vi "DBL to FXP Raw.vi"(7 "FXP Configuration":T1, 8 "error in (no error)":errorcluster, 10 "DBL Value":dbl) -> (0 "error out":errorcluster, 2 "Bool Data":bool[](array[boolean]))   [LabVIEW 2026, in "FPGA Register IO.lvlib"]
uses:
  FPGA Register IO.lvlib
  TypeDefs/FXP Configuration.ctl
  <vilib>/fxp/LVFixedPointRepBitsTypeDef.ctl
  <vilib>/fxp/LVFixedPointRepRangeTypeDef.ctl
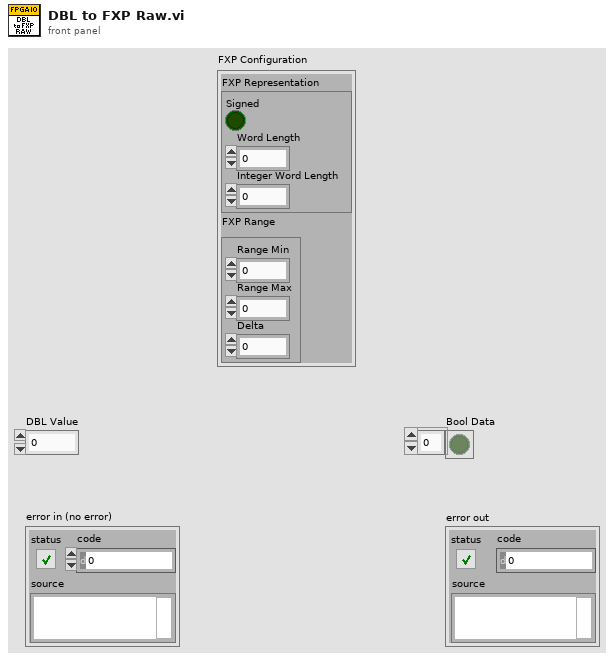
[diagram p1: front panel]
types:
  T1 = typedef "FPGA Register IO.lvlib/FXP Configuration.ctl" = cluster{"FXP Representation":T2, "FXP Range":T3}
  T2 = typedef "LVFixedPointRepBitsTypeDef.ctl" = cluster{"Signed":bool, "Word Length":u32, "Integer Word Length":i32}
  T3 = typedef "LVFixedPointRepRangeTypeDef.ctl" = cluster{"Range Min":dbl, "Range Max":dbl, "Delta":dbl}
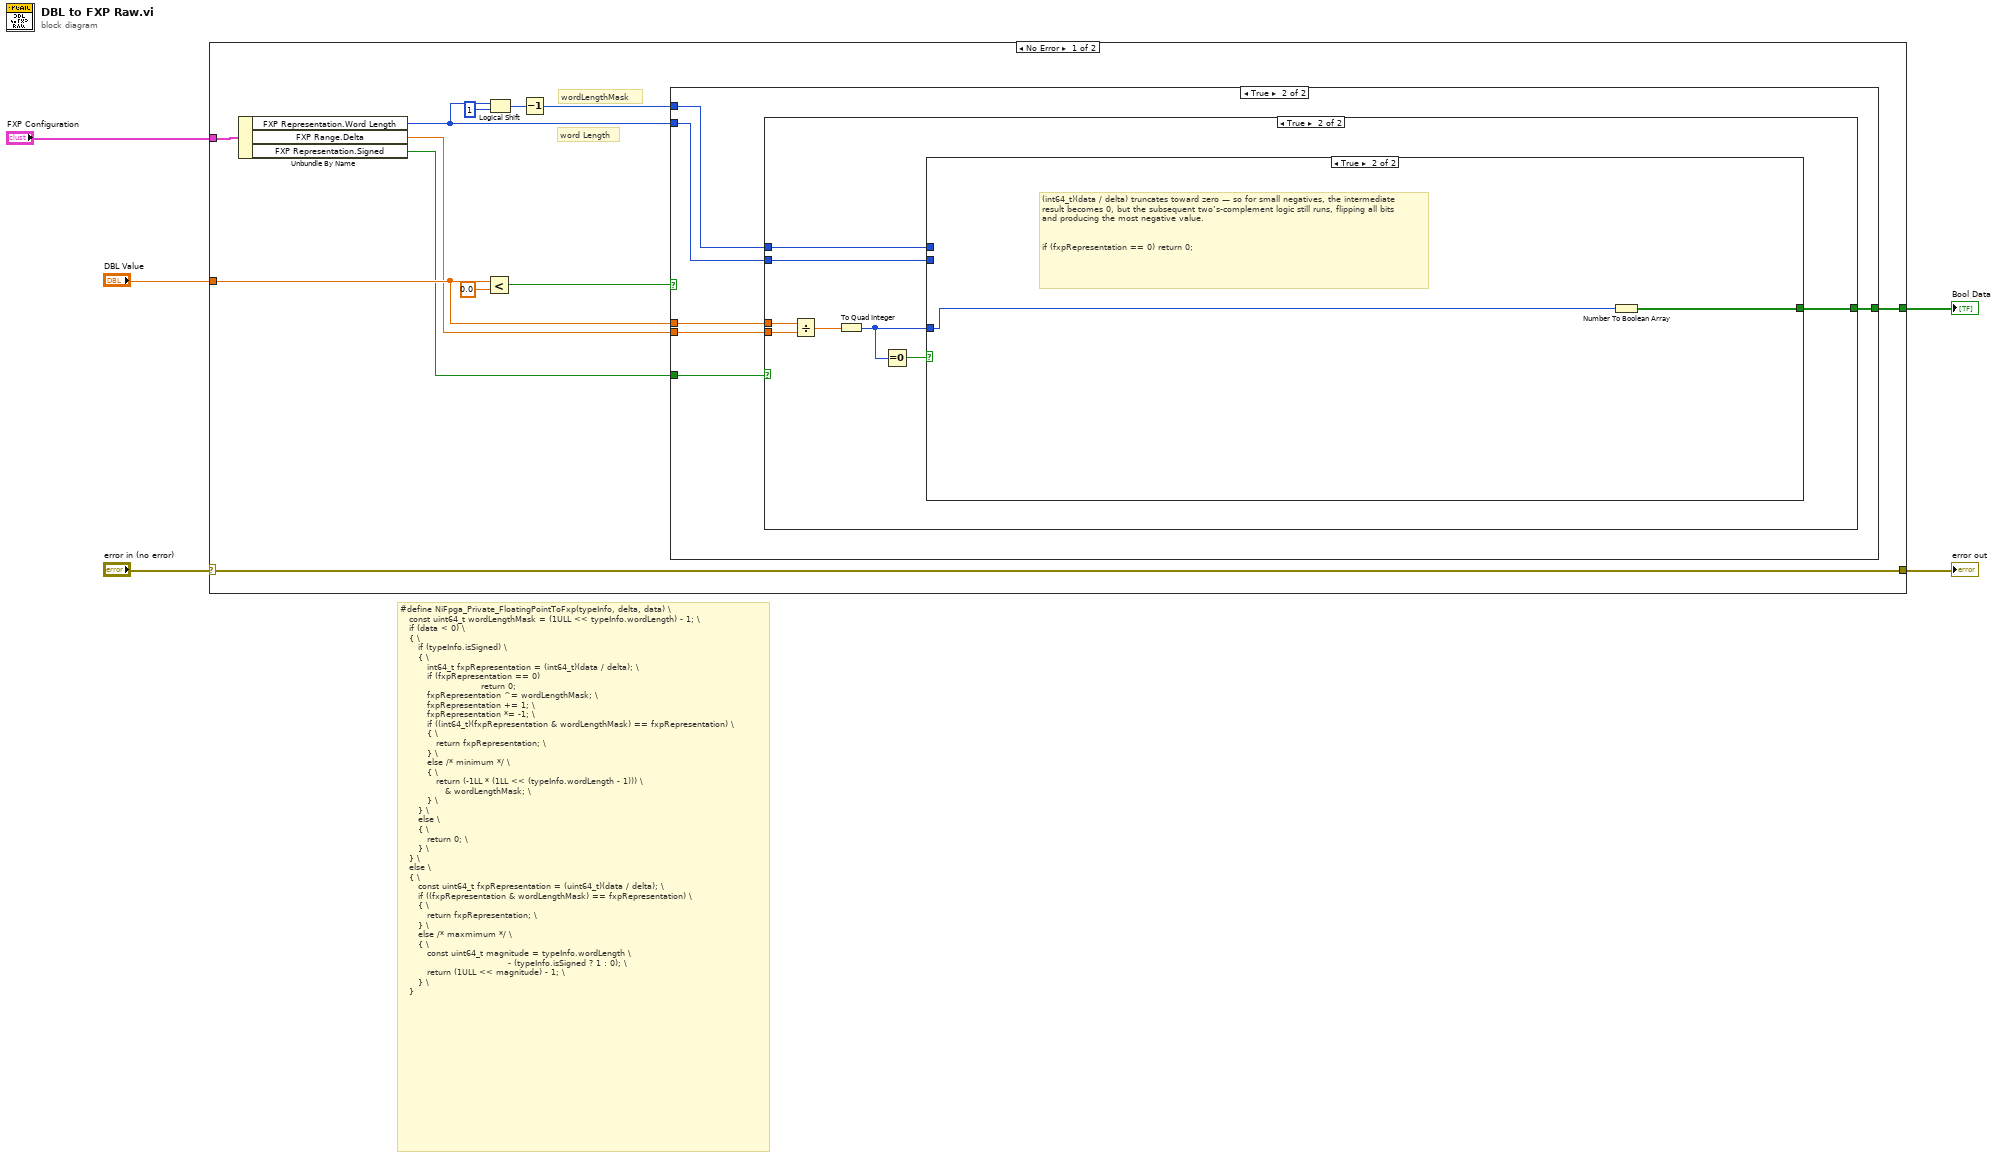
[diagram p0: block diagram]
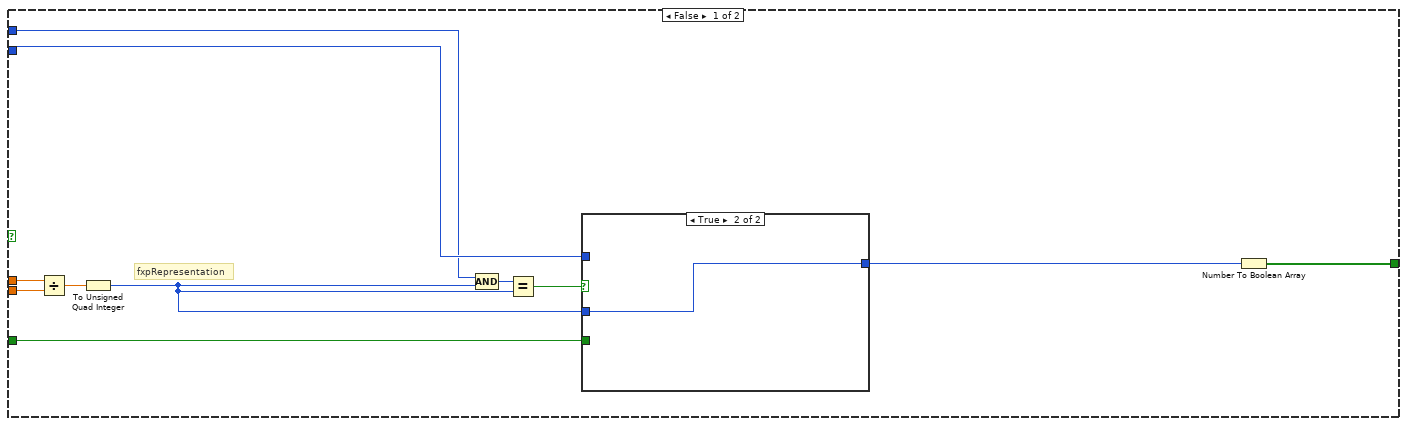
[diagram p2: hidden frame]
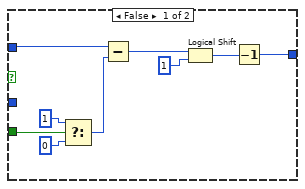
[diagram p3: hidden frame]
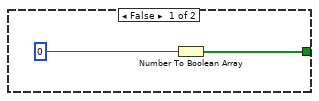
[diagram p4: hidden frame]
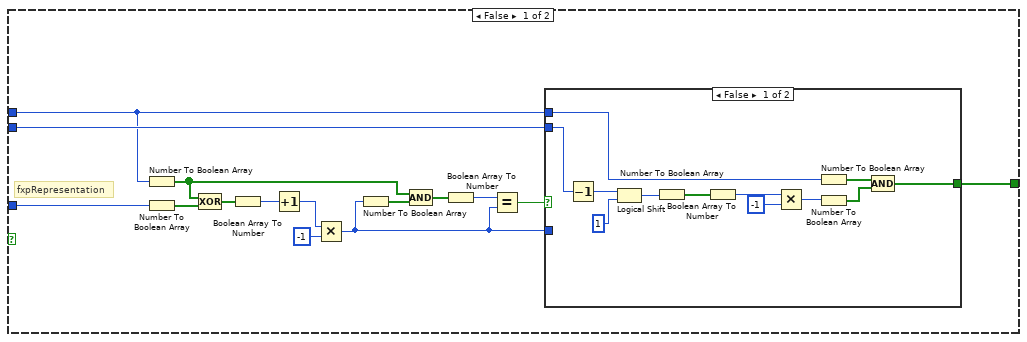
[diagram p5: hidden frame]
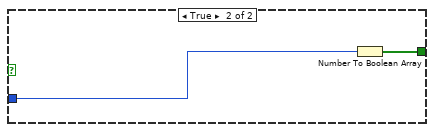
[diagram p6: hidden frame]
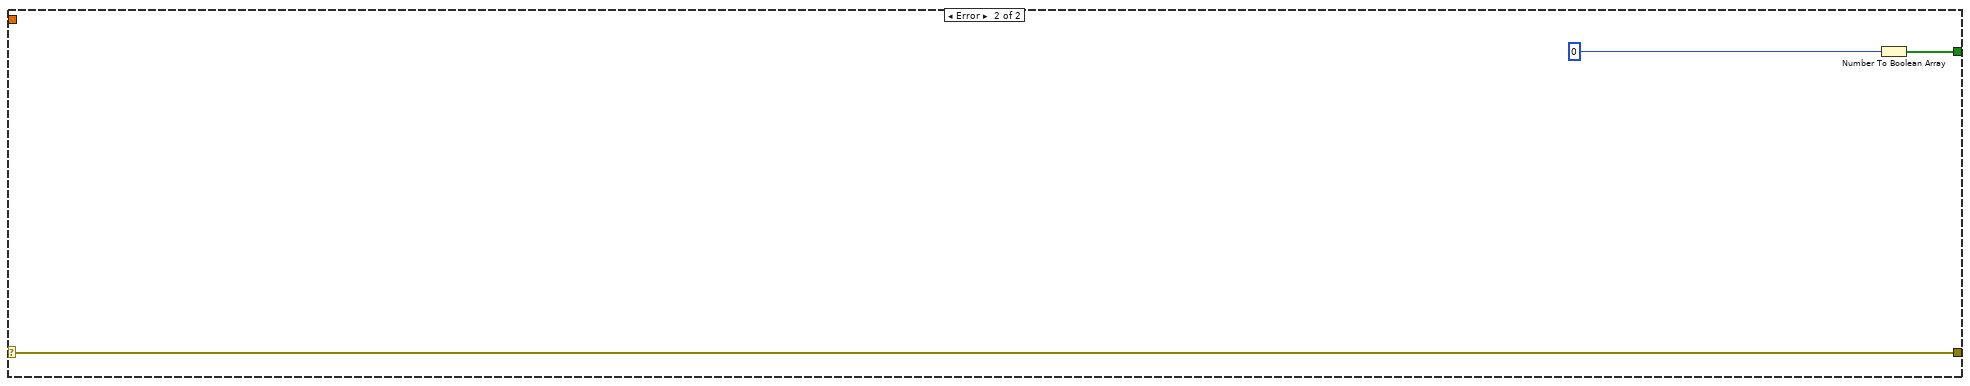
[diagram p7: hidden frame]
diagram:
  # "#define NiFpga_Private_FloatingPointToFxp(typeInfo, delta, data) \\\n   const uint64_t wordLengthMask = (1ULL << typeInfo.wordLength) - 1; \\\n   if (data < 0) \\\n   { \\\n      if (typeInfo.isSigned) \\\n      { \\\n         int64_t fxpRepresentation = (int64_t)(data / delta); \\\n         if (fxpRepresentation == 0)\n                           return 0;\n         fxpRepresentation ^= wordLengthMask; \\\n         fxpRepresentation += 1; \\\n         fxpRepresentation *= -1; \\\n         if ((int64_t)(fxpRepresentation & wordLengthMask) == fxpRepresentation) \\\n         { \\\n            return fxpRepresentation; \\\n         } \\\n         else /* minimum */ \\\n         { \\\n            return (-1LL * (1LL << (typeInfo.wordLength - 1))) \\\n               & wordLengthMask; \\\n         } \\\n      } \\\n      else \\\n      { \\\n         return 0; \\\n      } \\\n   } \\\n   else \\\n   { \\\n      const uint64_t fxpRepresentation = (uint64_t)(data / delta); \\\n      if ((fxpRepresentation & wordLengthMask) == fxpRepresentation) \\\n      { \\\n         return fxpRepresentation; \\\n      } \\\n      else /* maxmimum */ \\\n      { \\\n         const uint64_t magnitude = typeInfo.wordLength \\\n                                    - (typeInfo.isSigned ? 1 : 0); \\\n         return (1ULL << magnitude) - 1; \\\n      } \\\n   }"
  n1 = case shown="No Error" "error in (no error)" {
    selector: "error in (no error)" -> [w8 w88]
    tunnel: "FXP Configuration" -> [w12 _]
    tunnel: [w8 w88] -> w4
    tunnel: "DBL Value" -> [w11 _]
    tunnel: [w7 w87] -> w1
    frame No Error {
      # "word Length"
      # "wordLengthMask"
      n2 = Unbundle By Name(w12) -> ("FXP Representation.Word Length"=w6:u32, "FXP Range.Delta"=w10:dbl, "FXP Representation.Signed"=w9:bool)
      n3 = Less?(x=w11, y=0.0) -> (x < y?=w14:bool)
      n4 = Logical Shift(y=w6, x=u64 1) -> (x << y=w17:u64)
      n5 = Decrement(x=w17) -> (x-1=w13:u64)
      n6 = case shown="True" w14 {
        tunnel: w9 -> [w22 w44]
        tunnel: w11 -> [w28 w43]
        tunnel: w10 -> [w27 w42]
        tunnel: w6 -> [w23 w41]
        tunnel: w13 -> [w21 w40]
        tunnel: [w18 w39] -> w7
        frame False {
          # "fxpRepresentation"
          n7 = Divide(x=w28, y=w27) -> (x/y=w26:dbl)
          n8 = To Unsigned Quad Integer(1:w26) -> (0:w20:u64)
          n9 = Compound Arithmetic op=AND(w21, w20) -> (w25:u64)
          n10 = Equal?(x=w25, y=w20) -> (x = y?=w24:bool)
          n11 = case shown="True" w24 {
            tunnel: [w29 w38] -> w19
            tunnel: w23 -> [w34 _]
            tunnel: w22 -> [w37 _]
            tunnel: w20 -> [_ w38]
            frame False {
              n12 = Select(t=u32 1 ("word length"), s=w37, f=u32 0) -> (s? t:f=w33:u32)
              n13 = Subtract(x=w34, y=w33) -> (x-y=w32:u32)
              n14 = Logical Shift(y=w32, x=u64 1) -> (x << y=w30:u64)
              n15 = Decrement(x=w30) -> (x-1=w29:u64)
            }
            frame True {
            }
          }
          n16 = Number To Boolean Array(number=w19) -> (Boolean array=w18:bool[])
        }
        frame True {
          n17 = case shown="True" w44 {
            tunnel: w43 -> [_ w54]
            tunnel: w42 -> [_ w53]
            tunnel: w40 -> [_ w50]
            tunnel: w41 -> [_ w51]
            tunnel: [w46 w49] -> w39
            frame False {
              n18 = Number To Boolean Array(number=i64 0) -> (Boolean array=w46:bool[])
            }
            frame True {
              n19 = Divide(x=w54, y=w53) -> (x/y=w52:dbl)
              n20 = To Quad Integer(1:w52) -> (0:w48:i64)
              n21 = Equal To 0?(x=w48) -> (x = 0?=w47:bool)
              n22 = case shown="True" w47 {
                tunnel: w48 -> [w69 w85]
                tunnel: w51 -> [w60 _]
                tunnel: w50 -> [w56 _]
                tunnel: [w55 w84] -> w49
                frame False {
                  # "fxpRepresentation"
                  n23 = Number To Boolean Array(number=w56) -> (Boolean array=w64:bool[])
                  n24 = Number To Boolean Array(number=w69) -> (Boolean array=w68:bool[])
                  n25 = Compound Arithmetic op=XOR(w64, w68) -> (w67:bool[])
                  n26 = Boolean Array To Number(Boolean array=w67) -> (number=w66:i64)
                  n27 = Increment(x=w66) -> (x+1=w59:i64)
                  n28 = Multiply(x=w59, y=i64 -1) -> (x*y=w57:i64)
                  n29 = Number To Boolean Array(number=w57) -> (Boolean array=w63:bool[])
                  n30 = Compound Arithmetic op=AND(w64, w63) -> (w62:bool[])
                  n31 = Boolean Array To Number(Boolean array=w62) -> (number=w58:i64)
                  n32 = Equal?(x=w58, y=w57) -> (x = y?=w61:bool)
                  n33 = case shown="False" w61 {
                    tunnel: w60 -> [w79 _]
                    tunnel: w56 -> [w73 _]
                    tunnel: w57 -> [_ w83]
                    tunnel: [w70 w82] -> w55
                    frame False {
                      n34 = Decrement(x=w79) -> (x-1=w80:u32)
                      n35 = Logical Shift(y=w80, x=u64 1) -> (x << y=w78:u64)
                      n36 = Number To Boolean Array(number=w78) -> (Boolean array=w77:bool[])
                      n37 = Boolean Array To Number(Boolean array=w77) -> (number=w76:i64)
                      n38 = Multiply(x=w76, y=i64 -1) -> (x*y=w74:i64)
                      n39 = Number To Boolean Array(number=w73) -> (Boolean array=w72:bool[])
                      n40 = Number To Boolean Array(number=w74) -> (Boolean array=w71:bool[])
                      n41 = Compound Arithmetic op=AND(w72, w71) -> (w70:bool[])
                    }
                    frame True {
                      n42 = Number To Boolean Array(number=w83) -> (Boolean array=w82:bool[])
                    }
                  }
                }
                frame True {
                  # "(int64_t)(data / delta) truncates toward zero — so for small negatives, the intermediate result becomes 0, but the subsequent two’s-complement logic still runs, flipping all bits and producing the most negative value.\n\n\nif (fxpRepresentation == 0) return 0;"
                  n43 = Number To Boolean Array(number=w85) -> (Boolean array=w84:bool[])
                }
              }
            }
          }
        }
      }
    }
    frame Error {
      n44 = Number To Boolean Array(number=u64 0) -> (Boolean array=w87:bool[])
    }
  }
  "error out" <- w4
  "Bool Data" <- w1
